vi "Prepare VI for Parameterized Test.vi"(8 "error in":errorcluster, 11 "VI in":refnum<vi>) -> (0 "error out":errorcluster, 1 "Indicators":map{string, refnum<vi>}(c390), 2 "Controls":map{string, refnum<vi>}(c390), 3 "VI out":refnum<vi>)   [LabVIEW 2020, in "Approval Tests.lvlib"]
uses:
  Approval Tests.lvlib
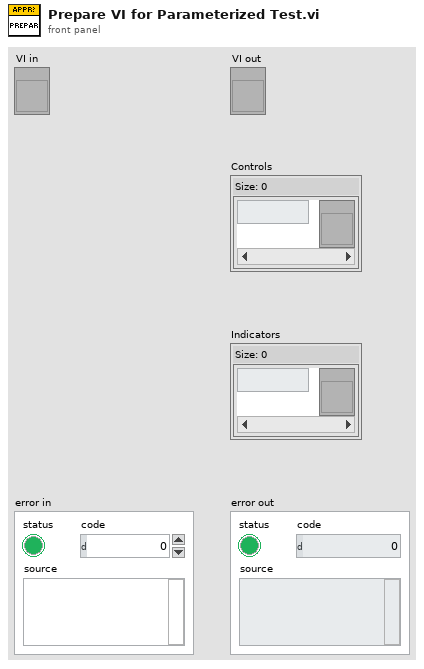
[diagram p1: front panel]
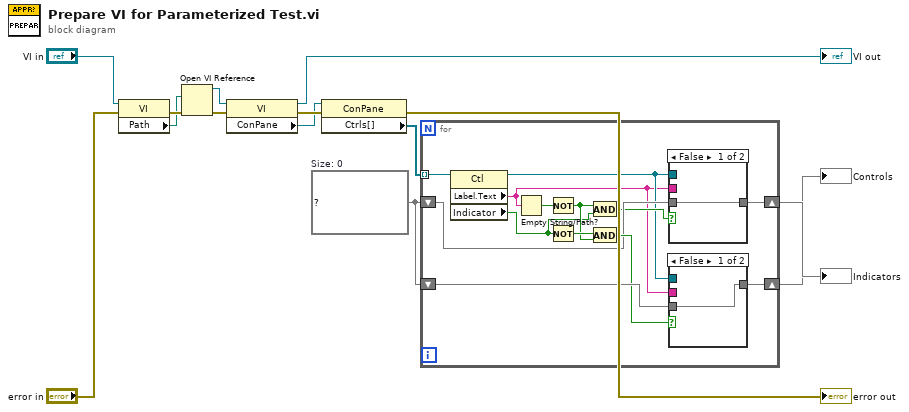
[diagram p0: block diagram]
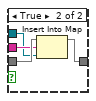
[diagram p2: hidden frame]
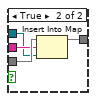
[diagram p3: hidden frame]
diagram:
  w5 = map{string, refnum<vi>} {}  # Size: 0
  n1 = property on="Property Node" class="VI"(reference="VI in", error in="error in") -> (error out=w10:errorcluster, "Path"=w3:path)  [unwired: 1 out]
  n2 = Open VI Reference(vi path=w3, error in (no error)=w10) -> (vi reference=w4:refnum<vi>, error out=w11:errorcluster)  [unwired: 4 in]
  n3 = property on="Property Node" class="VI"(reference=w4, error in=w11) -> (reference out=→"VI out":refnum<vi>, error out=w12:errorcluster, "ConPane"=w1:refnum<vi>)
  n4 = property on="Property Node" class="ConPane"(reference=w1, error in=w12) -> (error out=→"error out":errorcluster, "Ctrls[]"=w2:refnum<vi>[])  [unwired: 1 out]
  n5 = for {
    tunnel: w2 -> [w27] mode=indexing
    shift-right: [w25] -> w6
    shift-left: w5 -> [w26]
    shift-right: [w15] -> w7
    shift-left: w5 -> [w19]
    n6 = property on="Property Node" class="Ctl"(reference=w27) -> (reference out=w17:refnum<vi>, "Label.Text"=w16:string, "Indicator"=w20:bool)  [unwired: 1 in, 1 out]
    n7 = Empty String/Path?(string/path=w16) -> (empty?=w22:bool)
    n8 = Not(x=w22) -> (.not. x?=w21:bool)
    n9 = Not(x=w20) -> (.not. x?=w24:bool)
    n10 = And(x=w21, y=w20) -> (x .and. y?=w18:bool)
    n11 = And(x=w24, y=w21) -> (x .and. y?=w23:bool)
    n12 = case shown="False" w18 {
      tunnel: w19 -> [w28 w32]
      tunnel: [w28 w31] -> w15
      tunnel: w16 -> [_ w30]
      tunnel: w17 -> [_ w29]
      frame False {
      }
      frame True {
        n13 = Insert Into Map(map in=w32, key=w30, value=w29) -> (map out=w31:map{string, refnum<vi>})  [unwired: 2 out]
      }
    }
    n14 = case shown="False" w23 {
      tunnel: w26 -> [w33 w37]
      tunnel: [w33 w36] -> w25
      tunnel: w16 -> [_ w35]
      tunnel: w17 -> [_ w34]
      frame False {
      }
      frame True {
        n15 = Insert Into Map(map in=w37, key=w35, value=w34) -> (map out=w36:map{string, refnum<vi>})  [unwired: 2 out]
      }
    }
  }
  "Indicators" <- w7
  "Controls" <- w6
